vi "configureAcquisition.vi"(8 "error in (no error)":errorcluster, 11 "ICCameraAcquisitor in":refnum<class "ICCameraAcquisitor.lvclass">) -> (0 "error out":errorcluster, 3 "ICCameraAcquisitor out":refnum<class "ICCameraAcquisitor.lvclass">)   [LabVIEW 2011, in "Hardware.lvlib" / "Channels.lvlib" / "ICCameraAcquisitor.lvclass"]
uses:
  ICCameraAcquisitor.lvclass
  ICCameraAcquisitor.lvclass/ICCameraAcquisitor.ctl
panel:
  out "Device":string
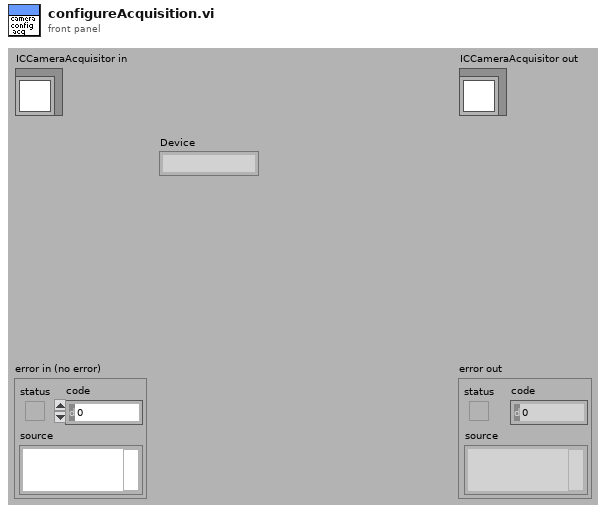
[diagram p1: front panel]
types:
  T1 = cluster{"Acquisition mode":dbl, "Readout Mode":dbl, "Gain":dbl}
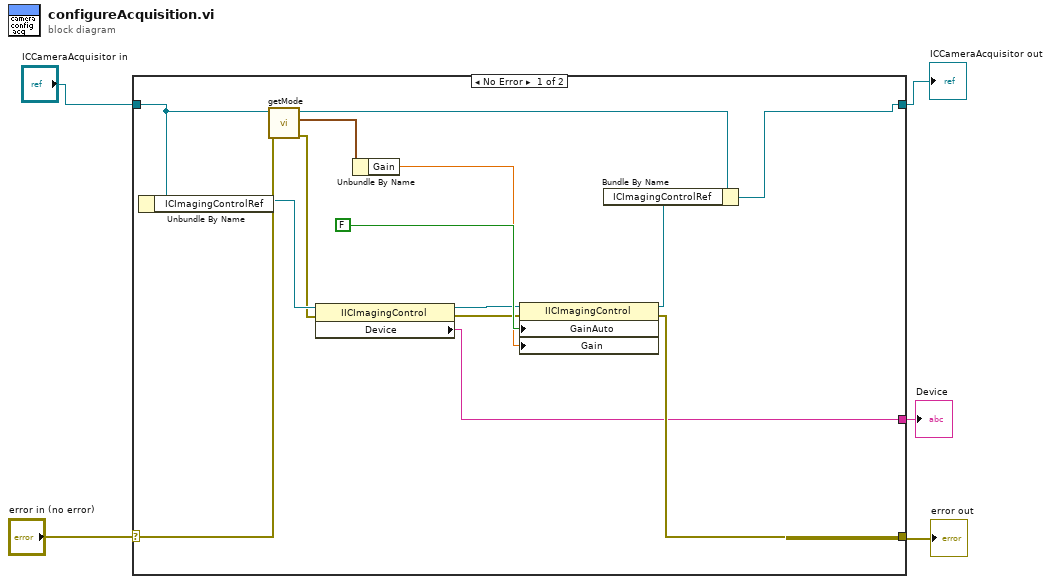
[diagram p0: block diagram]
diagram:
  n1 = case shown="No Error" "error in (no error)" {
    selector: "error in (no error)" -> [w18 w20]
    tunnel: "ICCameraAcquisitor in" -> [w19 w21]
    tunnel: [w13 w21] -> w3
    tunnel: [w12 w20] -> w2
    tunnel: [w6 _] -> w1
    frame No Error {
      n2 = Unbundle By Name(w19) -> ("ICImagingControlRef"=w11:refnum<k7>)
      n3 = call-dynamic "getMode.vi"("error in (no error)"=w18, "CameraAcquisitor.lvclass in"=w19) -> ("error out"=w10:errorcluster, "Mode"=w17:T1, "CameraAcquisitor.lvclass out"=w14:refnum<class "ICCameraAcquisitor.lvclass">)  [unwired: 7 in]
      n4 = property class="IICImagingControl"(reference=w11, error in=w10) -> (reference out=w9:refnum<k7>, error out=w8:errorcluster, "Device"=w6:string)
      n5 = Unbundle By Name(w17) -> ("Gain"=w15:dbl)
      n6 = property class="IICImagingControl"(reference=w9, error in=w8, "GainAuto"=FALSE, "Gain"=w15) -> (reference out=w7:refnum<k7>, error out=w12:errorcluster)
      n7 = Bundle By Name(cluster=w14, "ICImagingControlRef"=w7) -> (w13:refnum<class "ICCameraAcquisitor.lvclass">)
    }
    frame Error {
    }
  }
  "error out" <- w2
  "ICCameraAcquisitor out" <- w3
  "Device" <- w1
